vi "P Controller.vi"(2 "Kp":dbl=1.0, 3 "Setpoint":dbl, 4 "Process Variable":dbl) -> (0 "Output":dbl)   [LabVIEW 2013]
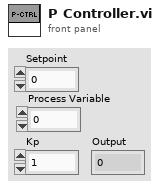
[diagram p1: front panel]
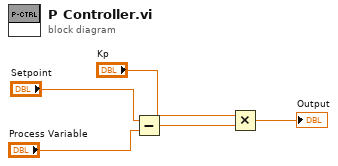
[diagram p0: block diagram]
diagram:
  n1 = Subtract(x="Setpoint", y="Process Variable") -> (x-y=w3:dbl)
  n2 = Multiply(x="Kp", y=w3) -> (x*y=→"Output":dbl)
